vi "Formular Edit.vi"(10 "Project":string, 11 "Identifier In":string[](array[string])) -> (2 "OK?":bool, 3 "Identifier In":string[](array[string]))   [LabVIEW 2020]
uses:
  <vilib>/Utility/miscctls.llb/LVRowAndColumnTypeDef.ctl
panel:
  out "ID Valid":bool
  in  "Parameter List":i32(listbox) caption="变量列表"
  in  "Calculate":bool
  in  "Unit":string caption="单位"
  out "Value":string caption="值"
  in  "Formular":string caption="公式"
  in  "Name":string caption="名称"
  in  "Identifier":string caption="标识符"
  in  "Cancle":bool
  in  "OK":bool
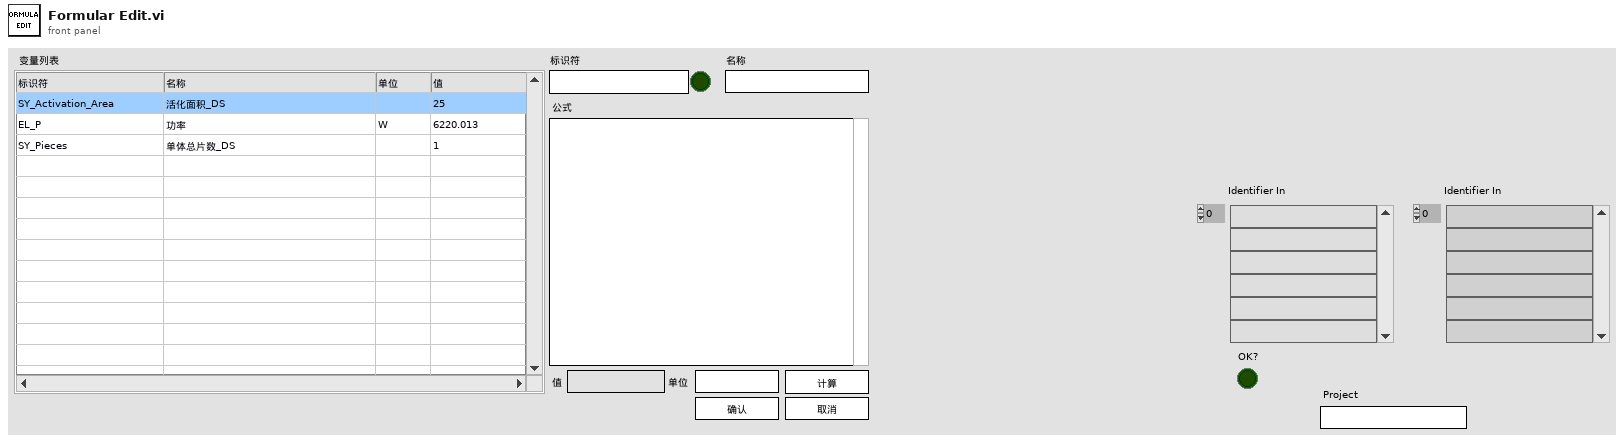
[diagram p1: front panel]
types:
  T1 = typedef "LVPoint32TypeDef.ctl" = cluster{"Horizontal":i32, "Vertical":i32}
  T2 = typedef "LVRowAndColumnTypeDef.ctl" = cluster{"Row":i32, "Column":i32}
  T3 = cluster{"Data":cluster{"ID":string, "Name":string, "Unit":string, "Value":string}[], "Project":string}
  T4 = cluster{"ID":string, "Name":string, "Unit":string, "Value":string}
  T5 = typedef "SDQ Data Type.ctl" = cluster{"CAN Length":string, "CAN Name":string, "CAN ID":string, "CAN Type":string, "Test Item":string, "Byte Order":string, "Instruction":string, "Control Type":string, "Group":string, "Offset":dbl, "Coefficient":dbl, "Write Enable":bool, "Lable Type":string, "Key?":string, "Set Value":string, "Upper":dbl, "Lower":dbl, "Unit":string, "Formula":string, "Test Item Type":string, "Length":i32, "Address":string, "Name":string, "Identifier":string, "Data Type":string, "Enumerate?":string, "Enumerate List":string, "Data":string, "Source":string}
  T6 = cluster{"ID":string, "Name":string, "Unit":string, "Value":string}[]
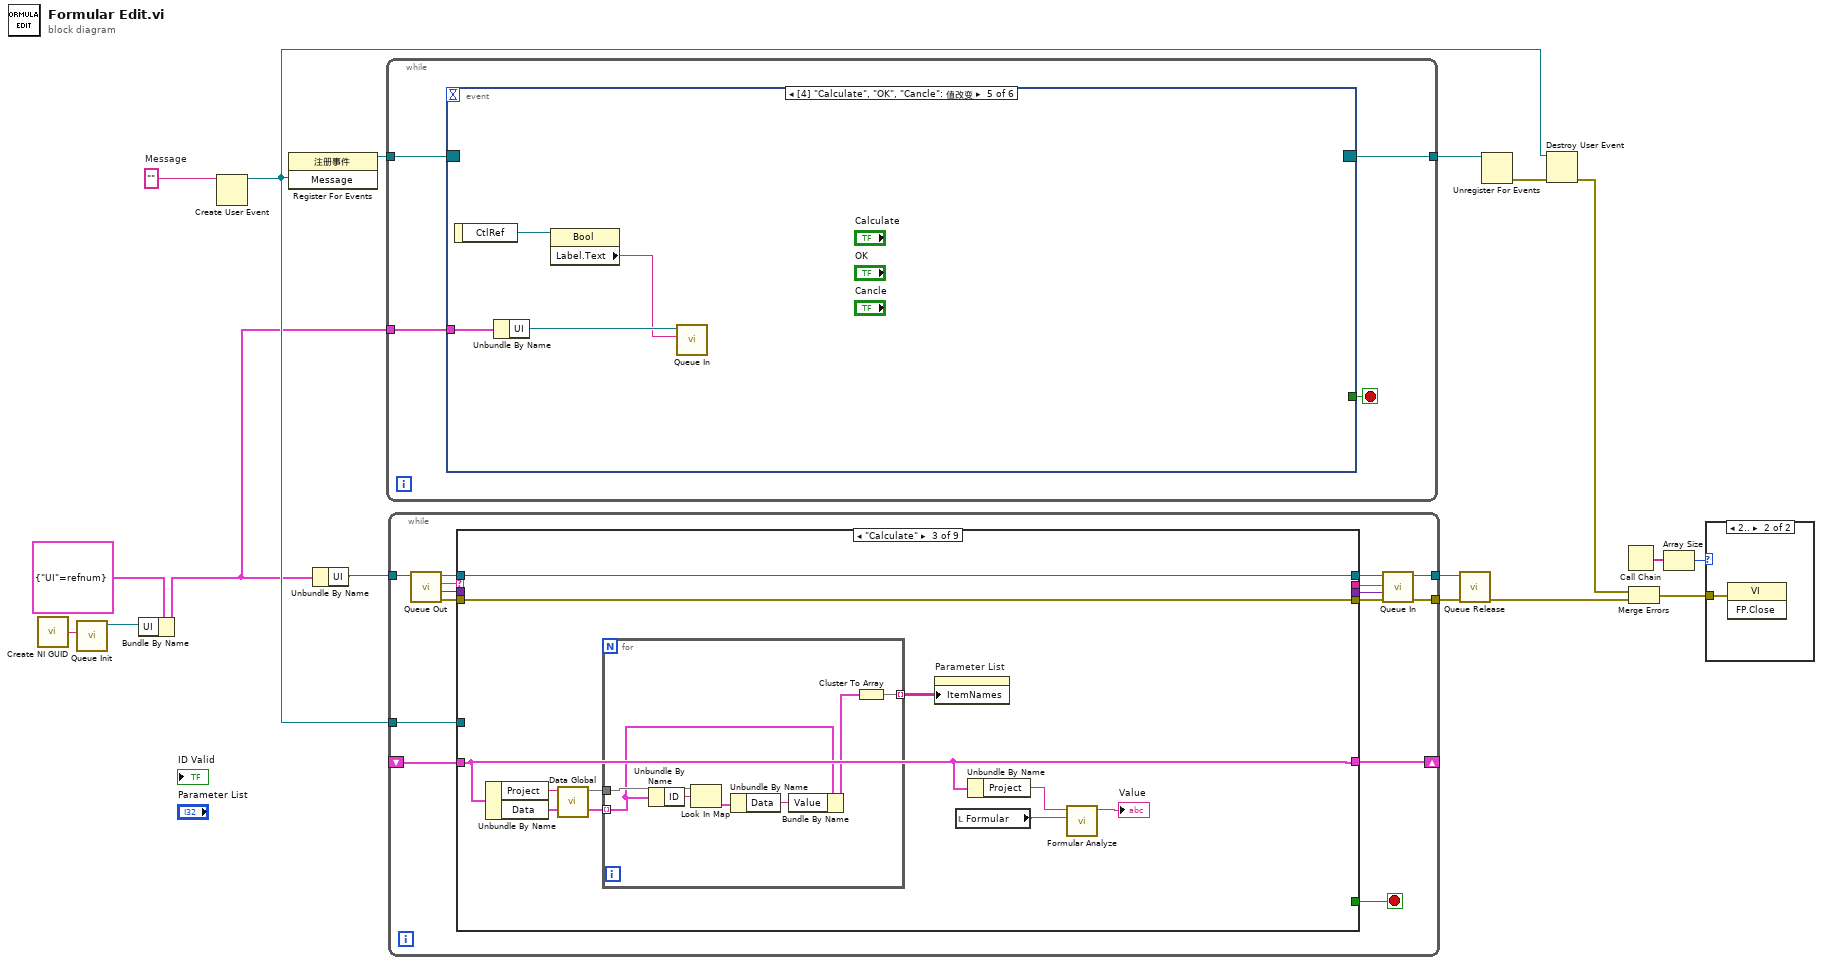
[diagram p0: block diagram]
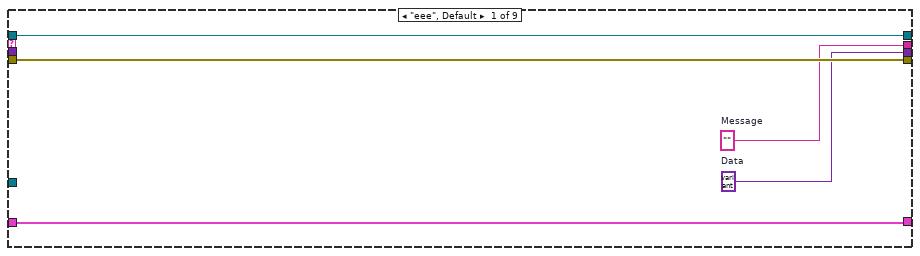
[diagram p3: hidden frame]
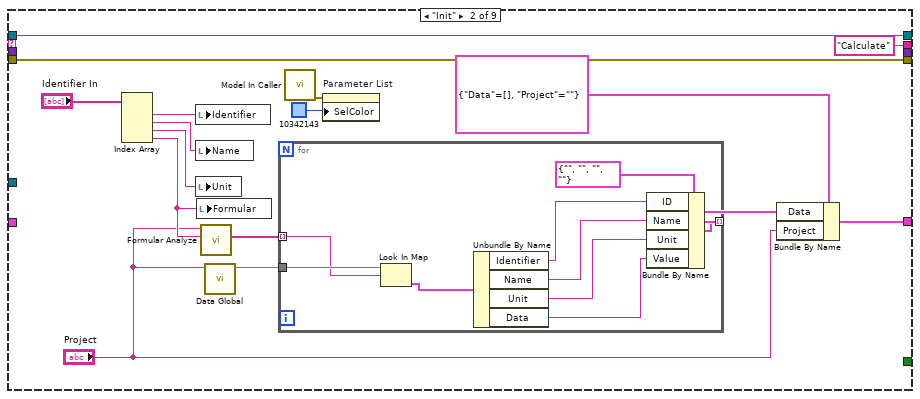
[diagram p4: hidden frame]
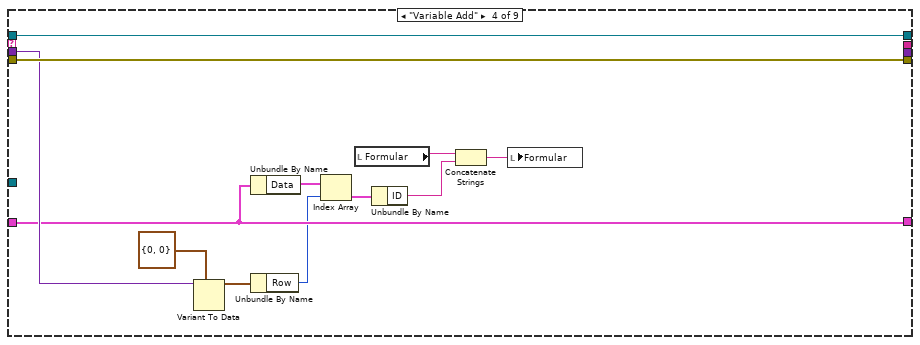
[diagram p5: hidden frame]
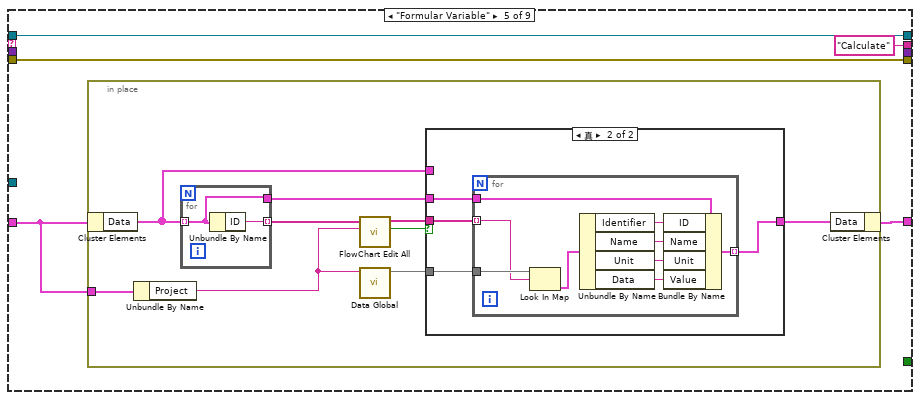
[diagram p6: hidden frame]
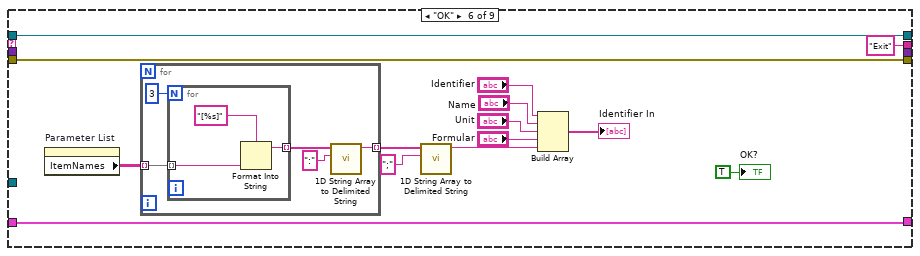
[diagram p8: hidden frame]
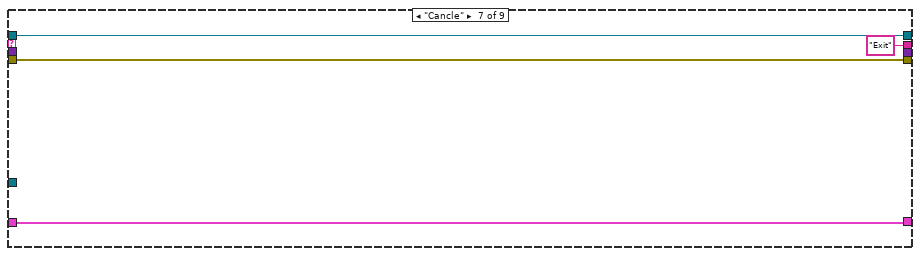
[diagram p9: hidden frame]
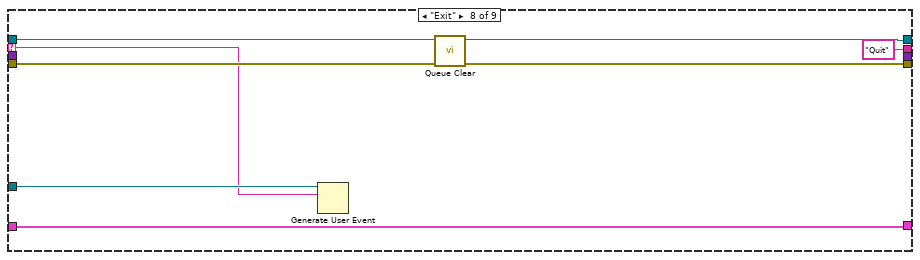
[diagram p10: hidden frame]
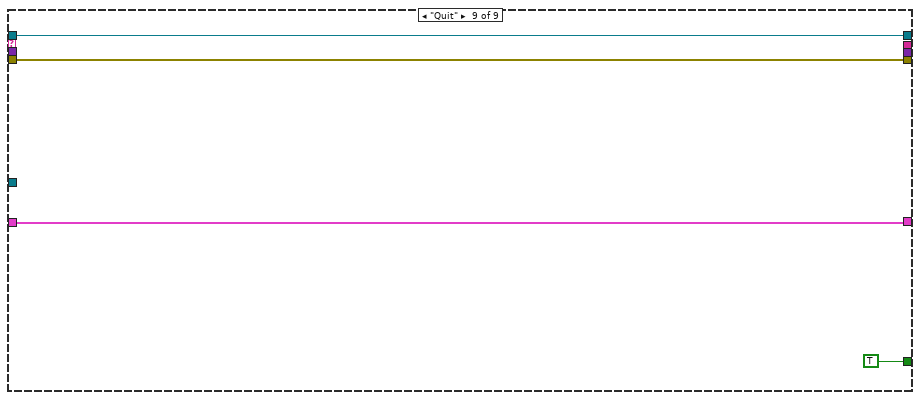
[diagram p11: hidden frame]
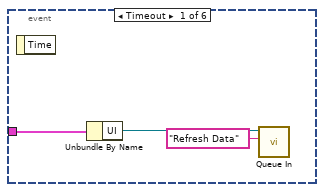
[diagram p12: hidden frame]
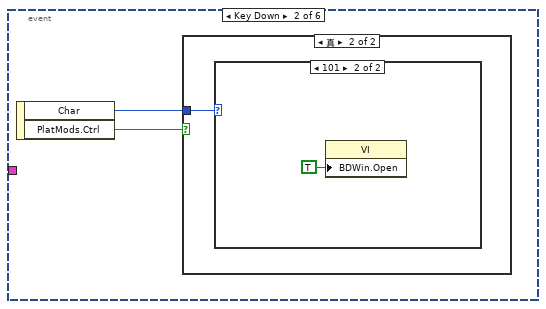
[diagram p13: hidden frame]
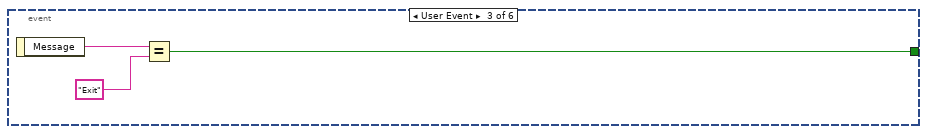
[diagram p16: hidden frame]
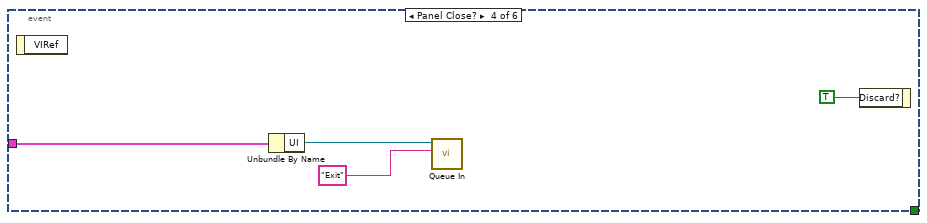
[diagram p17: hidden frame]
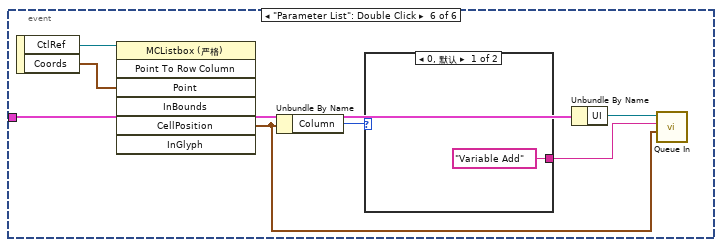
[diagram p18: hidden frame]
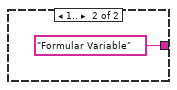
[diagram p19: hidden frame]
diagram:
  w5 = ""  # Message
  n1 = call <vilib>:"Create NI GUID.vi"() -> ("NI GUID"=w3:string)
  n2 = call "Queue Init.vi"("Queue Name"=w3) -> ("Queue Out"=w1:refnum<queue>)  [unwired: 8 in, 2 out]
  n3 = Bundle By Name(cluster=cluster{"UI":refnum<queue>} {"UI"=refnum} ("Queue Ref Out"), "UI"=w1) -> (w2:cluster{"UI":refnum<queue>})
  n4 = Create User Event(user event datatype=w5) -> (user event=w9:refnum<user-event>)  [unwired: 1 in, 1 out]
  n5 = register-events(w9) -> (reference out=w6:refnum<event-registration>)  [unwired: 2 in, 1 out]
  n6 = Unbundle By Name(w2) -> ("UI"=w12:refnum<queue>)
  n7 = while {
    tunnel: w6 -> [w21]
    tunnel: [w19] -> w7
    tunnel: w2 -> [w18]
    stop <- w20 stop-if-true
    n8 = event shown="[4] \"Calculate\", \"OK\", \"Cancle\": 值改变" {
      selector: w21 -> [_ _ _ _ _ _]
      dyn-events: [_ _ _ _ _ _] -> w19
      timeout: _ -> [_ _ _ _ _ _]
      tunnel: [_ _ w29 _ _ _] -> w20
      tunnel: w18 -> [w24 _ _ w34 w39 w46]
      event Timeout {
        n9 = event-data() -> ()  [unwired: 1 in, 1 out]
        n10 = Unbundle By Name(w24) -> ("UI"=w23:refnum<queue>)
        n11 = call "Queue In.vi"("Message"="Refresh Data", "Queue In"=w23) -> ()  [unwired: 8 in, 2 out]
      }
      event Key Down {
        n12 = event-data() -> ("Char"=w26:i16, "PlatMods.Ctrl"=w25:bool)  [unwired: 1 in]
        n13 = case shown="真" w25 {
          tunnel: w26 -> [_ w27]
          frame False {
          }
          frame True {
            n14 = case shown="101" w27 {
              frame 0, Default {
              }
              frame 101 {
                n15 = property class="VI"("BDWin.Open"=TRUE ("程序框图窗口:打开")) -> ()  [unwired: 2 in, 2 out]
              }
            }
          }
        }
      }
      event User Event {
        n16 = event-data() -> ("Message"=w31:string)  [unwired: 1 in]
        n17 = Equal?(x=w31, y="Exit") -> (x = y?=w29:bool)
      }
      event Panel Close? {
        n18 = event-data() -> ()  [unwired: 1 in, 1 out]
        n19 = Unbundle By Name(w34) -> ("UI"=w33:refnum<queue>)
        n20 = call "Queue In.vi"("Message"="Exit", "Queue In"=w33) -> ()  [unwired: 8 in, 2 out]
        n21 = event-data("Discard?"=TRUE ("放弃？")) -> ()  [unwired: 1 in, 1 out]
      }
      event "Calculate", "OK", "Cancle": Value Change {
        n22 = event-data() -> ("CtlRef"=w37:refnum<vi>)  [unwired: 1 in]
        n23 = Unbundle By Name(w39) -> ("UI"=w38:refnum<queue>)
        n24 = property class="Bool"(reference=w37) -> ("Label.Text"=w36:string)  [unwired: 1 in, 2 out]
        n25 = call "Queue In.vi"("Message"=w36, "Queue In"=w38) -> ()  [unwired: 8 in, 2 out]
      }
      event "Parameter List": Double Click {
        n26 = event-data() -> ("CtlRef"=w43:refnum<vi>, "Coords"=w42:T1)  [unwired: 1 in]
        n27 = invoke class="MCListbox (严格)" method="Point To Row Column"(reference=w43, "Point"=w42) -> ("CellPosition"=w40:T2)  [unwired: 5 in, 6 out]
        n28 = Unbundle By Name(w40) -> ("Column"=w41:i32)
        n29 = case shown="0, 默认" w41 {
          tunnel: ["Variable Add" ("Message") "Formular Variable" ("Message")] -> w44
          frame 0, Default {
          }
          frame 1.. {
          }
        }
        n30 = Unbundle By Name(w46) -> ("UI"=w45:refnum<queue>)
        n31 = call "Queue In.vi"("Data"=w40, "Message"=w44, "Queue In"=w45) -> ()  [unwired: 7 in, 2 out]
      }
    }
  }
  n32 = while {
    tunnel: w12 -> [w58]
    tunnel: [w55] -> w10
    tunnel: [w54] -> w11
    tunnel: w9 -> [w62]
    shift-right: [w50] -> _
    shift-left: _ -> [w49]
    stop <- w63 stop-if-true
    n33 = call "Queue Out.vi"("Queue In"=w58) -> ("error out"=w61:errorcluster, "Data"=w59:variant, "Message"=w60:string, "Queue Out"=w57:refnum<queue>)  [unwired: 6 in, 1 out]
    n34 = case shown="\"Calculate\"" w60 {
      selector: w60 -> [_ _ _ _ _ _ _ w180 _]
      tunnel: w57 -> [w68 w84 w103 w122 w127 w166 w178 w184 w189]
      tunnel: w61 -> [w67 w83 w102 w121 w126 w165 w177 w182 w190]
      tunnel: [w68 w84 w103 w122 w127 w166 w178 w183 w189] -> w56
      tunnel: [w67 w83 w102 w121 w126 w165 w177 w181 w190] -> w53
      tunnel: [w66 "Calculate" ("Message") _ _ "Calculate" ("Message") "Exit" ("Message") "Exit" ("Message") "Quit" _] -> w52
      tunnel: [_ _ _ _ _ _ _ _ TRUE] -> w63
      tunnel: w62 -> [_ _ _ _ _ _ _ w186 _]
      tunnel: [w65 _ _ _ _ _ _ _ _] -> w51
      tunnel: w59 -> [_ _ _ w120 _ _ _ _ _]
      tunnel: [w64 w75 w95 w117 w125 w162 w175 w179 w187] -> w50
      tunnel: w49 -> [w64 _ w95 w117 w123 w162 w175 w179 w187]
      frame "eee", Default {
        w65 = variant  # Data
        w66 = ""  # Message
      }
      frame "Init" {
        n35 = Index Array(array="Identifier In") -> (element #1=w79:string, element #2=w78:string, element #3=w77:string, element #4=w72:string)  [unwired: 4 in]
        n36 = local write "Identifier"(w79) -> ()
        n37 = local write "Name"(w78) -> ()
        n38 = local write "Unit"(w77) -> ()
        n39 = local write "Formular"(w72) -> ()
        n40 = call "Formular Analyze.vi"("Formular"=w72, "Project"="Project") -> ("Parameter"=w70:string[])  [unwired: 5 in, 4 out]
        n41 = call "Data Global.vi"("Name"="Project") -> ("Data Out"=w69:map{string, T5})  [unwired: 7 in, 3 out]
        n42 = for {
          tunnel: [w92] -> w81 mode=indexing
          tunnel: w70 -> [w90] mode=indexing
          tunnel: w69 -> [w91]
          n43 = Look In Map(map=w91, key=w90) -> (value=w89:T5)  [unwired: 1 in, 1 out]
          n44 = Unbundle By Name(w89) -> ("Identifier"=w88:string, "Name"=w87:string, "Unit"=w86:string, "Data"=w85:string)
          n45 = Bundle By Name(cluster=T4 {"ID"="", "Name"="", "Unit"="", "Value"=""} ("簇"), "ID"=w88, "Name"=w87, "Unit"=w86, "Value"=w85) -> (w92:T4)
        }
        n46 = call "Model In Caller.vi"() -> ("error out"=w74:errorcluster)  [unwired: 11 in]
        n47 = property on="Parameter List" class="MCListbox (严格)"(error in=w74, "SelColor"=u32 10342143 ("选择颜色")) -> ()  [unwired: 1 in, 2 out]
        n48 = Bundle By Name(cluster=T3 {"Data"=[], "Project"=""}, "Data"=w81, "Project"="Project") -> (w75:T3)
      }
      frame "Calculate" {
        n49 = Unbundle By Name(w95) -> ("Project"=w99:string, "Data"=w100:T6)
        n50 = call "Data Global.vi"("Name"=w99) -> ("Data Out"=w98:map{string, T5})  [unwired: 7 in, 3 out]
        n51 = for {
          tunnel: w100 -> [w106] mode=indexing
          tunnel: [w110] -> w101 mode=indexing
          tunnel: w98 -> [w108]
          n52 = Unbundle By Name(w106) -> ("ID"=w107:string)
          n53 = Look In Map(map=w108, key=w107) -> (value=w105:T5)  [unwired: 1 in, 1 out]
          n54 = Unbundle By Name(w105) -> ("Data"=w104:string)
          n55 = Bundle By Name(cluster=w106, "Value"=w104) -> (w109:T4)
          n56 = Cluster To Array(cluster=w109) -> (array=w110:string[])
        }
        n57 = property on="Parameter List" class="MCListbox (严格)"("ItemNames"=w101) -> ()  [unwired: 2 in, 2 out]
        n58 = local read "Formular"() -> (w97:string)
        n59 = Unbundle By Name(w95) -> ("Project"=w94:string)
        n60 = call "Formular Analyze.vi"("Formular"=w97, "Project"=w94) -> ("Result"=→"Value":string)  [unwired: 5 in, 4 out]
      }
      frame "Variable Add" {
        n61 = Variant To Data(type=T2 {"Row"=0, "Column"=0} ("单元格位置"), Variant=w120) -> (data=w118:T2)  [unwired: 1 in, 1 out]
        n62 = Unbundle By Name(w117) -> ("Data"=w116:T6)
        n63 = Unbundle By Name(w118) -> ("Row"=w115:i32)
        n64 = Index Array(array=w116, index=w115) -> (element=w114:T4)
        n65 = local read "Formular"() -> (w113:string)
        n66 = Unbundle By Name(w114) -> ("ID"=w112:string)
        n67 = Concatenate Strings(w113, w112) -> (w111:string)
        n68 = local write "Formular"(w111) -> ()
      }
      frame "Formular Variable" {
        n69 = in-place {
          in-place-border: w123 -> [w129]
          n70 = in-place-cluster #1(w123) -> ("Data"=w130:T6)
          n71 = Unbundle By Name(w129) -> ("Project"=w128:string)
          n72 = for {
            tunnel: w130 -> [w151] mode=indexing
            tunnel: [w152] -> w136 mode=indexing
            tunnel: [w151] -> w132
            n73 = Unbundle By Name(w151) -> ("ID"=w152:string)
          }
          n74 = call "FlowChart Edit All.vi"("Name"=w128, "Identifier In"=w136) -> ("OK？"=w134:bool, "Identifiers Out"=w133:string[])  [unwired: 8 in]
          n75 = call "Data Global.vi"("Name"=w128) -> ("Data Out"=w135:map{string, T5})  [unwired: 7 in, 3 out]
          n76 = case shown="真" w134 {
            tunnel: w135 -> [_ w141]
            tunnel: w133 -> [_ w140]
            tunnel: w132 -> [_ w139]
            tunnel: [w137 w138] -> w131
            tunnel: w130 -> [w137 _]
            frame False {
            }
            frame True {
              n77 = for {
                tunnel: w141 -> [w150]
                tunnel: w140 -> [w149] mode=indexing
                tunnel: w139 -> [w147]
                tunnel: [w142] -> w138 mode=indexing
                n78 = Look In Map(map=w150, key=w149) -> (value=w148:T5)  [unwired: 1 in, 1 out]
                n79 = Unbundle By Name(w148) -> ("Identifier"=w146:string, "Name"=w143:string, "Unit"=w144:string, "Data"=w145:string)
                n80 = Bundle By Name(cluster=w147, "ID"=w146, "Name"=w143, "Unit"=w144, "Value"=w145) -> (w142:T4)
              }
            }
          }
          n81 = in-place-cluster #1("Data"=w131) -> (w125:T3)
        }
      }
      frame "OK" {
        n82 = property on="Parameter List" class="MCListbox (严格)"() -> ("ItemNames"=w159:string[][])  [unwired: 2 in, 2 out]
        n83 = for {
          tunnel: w159 -> [w171] mode=indexing
          tunnel: [w168] -> w160 mode=indexing
          n84 = for {
            N: 3 -> [_]
            tunnel: w171 -> [w173] mode=indexing
            tunnel: [w172] -> w170 mode=indexing
            n85 = Format Into String(format string="[%s]" ("格式字符串"), w173) -> (resulting string=w172:string)  [unwired: 2 in, 1 out]
          }
          n86 = call <vilib>:"1D String Array to Delimited String.vi"("delimiter"=":", "string array"=w170) -> ("delimited string"=w168:string)  [unwired: 9 in]
        }
        n87 = call <vilib>:"1D String Array to Delimited String.vi"("delimiter"=";", "string array"=w160) -> ("delimited string"=w161:string)  [unwired: 9 in]
        n88 = Build Array("Identifier", "Name", "Unit", "Formular", w161) -> (→"Identifier In":string[])
        "OK?" <- TRUE ("OK?")
      }
      frame "Cancle" {
      }
      frame "Exit" {
        n89 = Generate User Event(user event=w186, event data cluster=w180) -> ()  [unwired: 2 in, 2 out]
        n90 = call "Queue Clear.vi"("error in (no error)"=w182, "Queue In"=w184) -> ("error out"=w181:errorcluster, "Queue Out"=w183:refnum<queue>)  [unwired: 8 in]
      }
      frame "Quit" {
      }
    }
    n91 = call "Queue In.vi"("error in (no error)"=w53, "Data"=w51, "Message"=w52, "Queue In"=w56) -> ("error out"=w54:errorcluster, "Queue Out"=w55:refnum<queue>)  [unwired: 6 in]
  }
  n92 = call "Queue Release.vi"("error in (no error)"=w11, "Queue In"=w10) -> ("error out"=w14:errorcluster)  [unwired: 9 in]
  n93 = Unregister For Events(event registration refnum=w7) -> (error out=w8:errorcluster)  [unwired: 1 in]
  n94 = Destroy User Event(user event=w9, error in=w8) -> (error out=w13:errorcluster)
  n95 = Call Chain() -> (call chain=w16:string[])
  n96 = Merge Errors(w13, w14) -> (w15:errorcluster)
  n97 = Array Size(array=w16) -> (size(s)=w17:i32)
  n98 = case shown="2.." w17 {
    tunnel: w15 -> [_ w191]
    frame 0, Default {
    }
    frame 2.. {
      n99 = invoke class="VI" method="FP.Close"(error in=w191) -> ()  [unwired: 2 in, 3 out]
    }
  }
